vi "Login.vi"() -> ()   [LabVIEW 2020]
uses:
  <vilib>/httpClient/LabVIEWHTTPClient.lvlib
panel:
  out "Error Out":errorcluster
  in  "Error In":errorcluster
  in  "Visibility":bool
  in  "Login":bool
  in  "Clear":bool
  in  "Password":string
  in  "Username":string
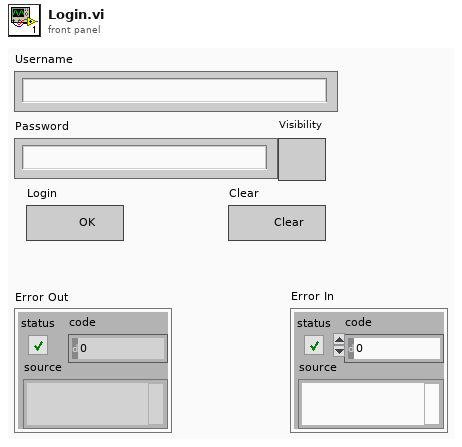
[diagram p1: front panel]
types:
  T1 = typedef "LabVIEWHTTPClient.lvlib/ClientHandle.ctl" = refnum<k1>
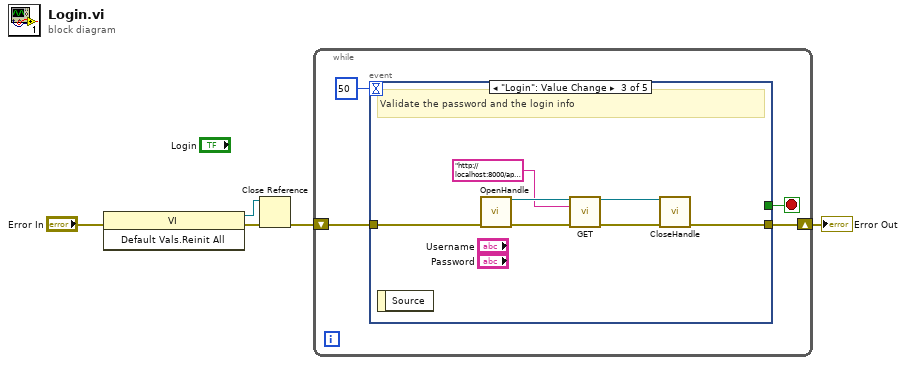
[diagram p0: block diagram]
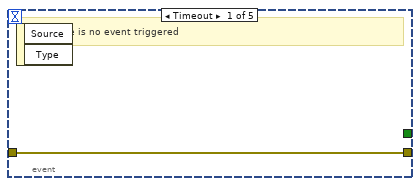
[diagram p2: hidden frame]
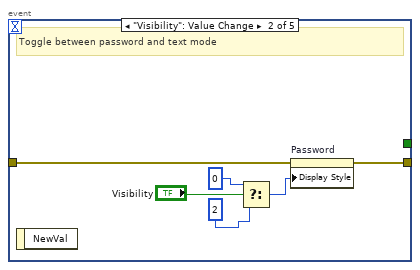
[diagram p3: hidden frame]
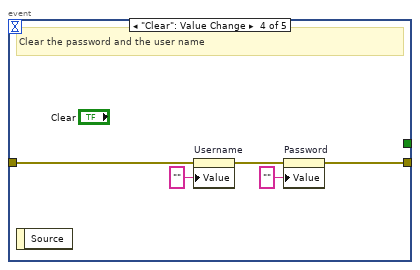
[diagram p4: hidden frame]
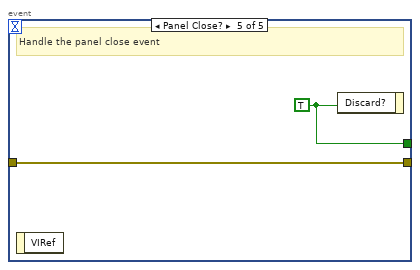
[diagram p5: hidden frame]
diagram:
  n1 = invoke class="VI" method="Default Vals.Reinit All"(error in="Error In") -> (reference out=w1:refnum<vi>, error out=w3:errorcluster)  [unwired: 2 in, 1 out]
  n2 = Close Reference(reference=w1, error in (no error)=w3) -> (error out=w2:errorcluster)
  n3 = while {
    shift-right: [w6] -> w4
    shift-left: w2 -> [w7]
    stop <- w8 stop-if-true
    n4 = event shown="[2] \"Login\": Value Change" {
      selector: _ -> [_ _ _ _ _]
      dyn-events: _ -> [_ _ _ _ _]
      timeout: 50 -> [_ _ _ _ _]
      tunnel: [_ _ _ _ w30] -> w8
      tunnel: [w10 w15 w21 w25 w29] -> w6
      tunnel: w7 -> [w10 w16 w23 w28 w29]
      event Timeout {
        # "When there is no event triggered"
        n5 = event-data() -> ()  [unwired: 1 in, 2 out]
      }
      event "Visibility": Value Change {
        # "Toggle between password and text mode"
        n6 = event-data() -> ()  [unwired: 1 in, 1 out]
        n7 = Select(t=u32 0, s="Visibility", f=u32 2) -> (s? t:f=w11:u32)
        n8 = property on="Password" class="Str"(error in=w16, "Display Style"=w11) -> (error out=w15:errorcluster)  [unwired: 1 in, 1 out]
      }
      event "Login": Value Change {
        # "Validate the password and the login info"
        n9 = event-data() -> ()  [unwired: 1 in, 1 out]
        n10 = call <vilib>:"OpenHandle.vi"("error in (no error)"=w23) -> ("client handle out"=w19:T1, "error out"=w22:errorcluster)  [unwired: 13 in]
        n11 = call <vilib>:"GET.vi"("client handle"=w19, "url"="http://localhost:8000/api/auth/user", "error in (no error)"=w22) -> ("client handle out"=w18:T1, "error out"=w20:errorcluster)  [unwired: 9 in, 2 out]
        n12 = call <vilib>:"CloseHandle.vi"("client handle"=w18, "error in (no error)"=w20) -> ("error out"=w21:errorcluster)  [unwired: 13 in]
      }
      event "Clear": Value Change {
        # "Clear the password and the user name"
        n13 = event-data() -> ()  [unwired: 1 in, 1 out]
        n14 = property on="Username" class="Str"(error in=w28, "Value"="" ("Username")) -> (error out=w27:errorcluster)  [unwired: 1 in, 1 out]
        n15 = property on="Password" class="Str"(error in=w27, "Value"="" ("Password")) -> (error out=w25:errorcluster)  [unwired: 1 in, 1 out]
      }
      event Panel Close? {
        w30 = TRUE
        # "Handle the panel close event"
        n16 = event-data() -> ()  [unwired: 1 in, 1 out]
        n17 = event-data("Discard?"=w30) -> ()  [unwired: 1 in, 1 out]
      }
    }
  }
  "Error Out" <- w4
